vi "GPS_file_append.vi"(8 "Alt":string[](array[string]), 9 "Lng":string[](array[string]), 10 "Lat":string[](array[string]), 11 "input cluster":T1={"System"={"Active"=FALSE, "Exit"=FALSE, "Command wait"="", "Status_Time"=0, "Time_GPS"=0}, "Stepper Motor"={"Connection Reference"="", "Valid Connection"=FALSE, "Speed"=15}, "Camera Data"={"Image path"=path "", "Filenames"=[], "Filenames queue"=[]}, "Core"={"Close Panel on Exit?"=FALSE, "Current VI Reference"=refnum}} {"Stepper Motor"."Speed" scale=0.0..30.0}) -> (2 "Data":string[][](array[string]), 3 "Filenames queue":string[](array[string]))   [LabVIEW 2019]
uses:
  System Data.ctl
  Stepper Data.ctl
  Camera Data.ctl
  <vilib>/Utility/file.llb/Write Delimited Spreadsheet (string).vi
  <vilib>/Utility/file.llb/Read Delimited Spreadsheet (string).vi
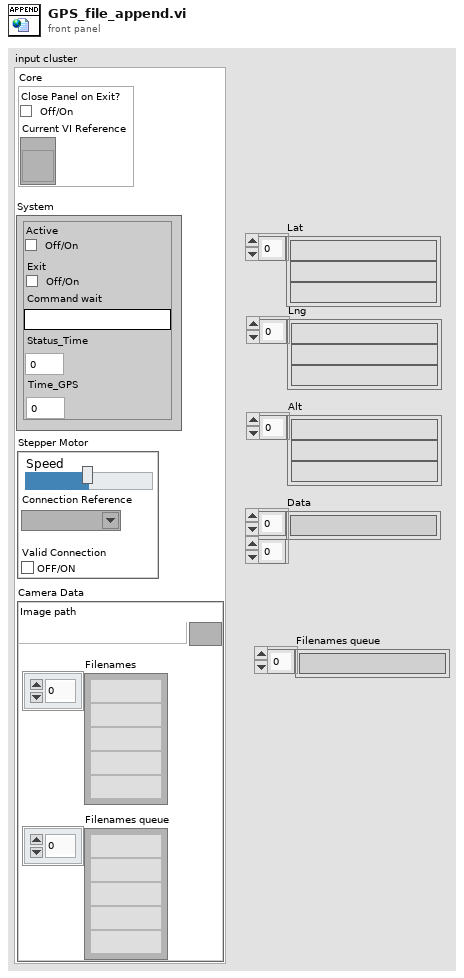
[diagram p1: front panel]
types:
  T1 = typedef "System Data.ctl" = cluster{"System":cluster{"Active":bool, "Exit":bool, "Command wait":string, "Status_Time":i32, "Time_GPS":i32}, "Stepper Motor":T2, "Camera Data":T3, "Core":cluster{"Close Panel on Exit?":bool, "Current VI Reference":refnum<vi>}}
  T2 = typedef "Stepper Data.ctl" = cluster{"Connection Reference":refnum<visa-resource-name>, "Valid Connection":bool, "Speed":i32}
  T3 = typedef "Camera Data.ctl" = cluster{"Image path":path, "Filenames":string[], "Filenames queue":string[]}
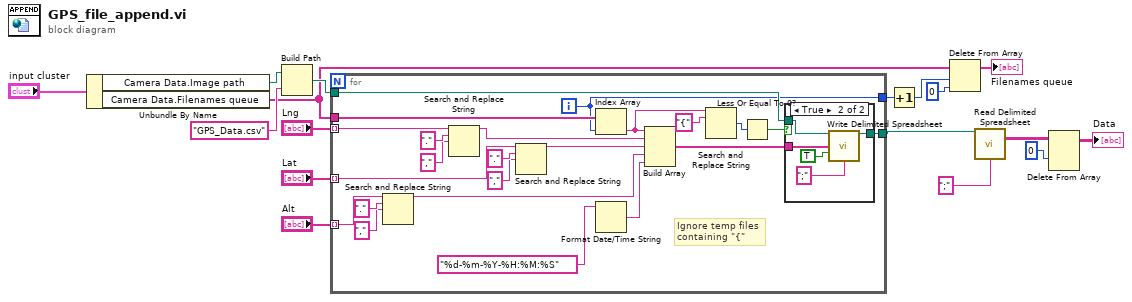
[diagram p0: block diagram]
diagram:
  n1 = Unbundle By Name("input cluster") -> ("Camera Data.Image path"=w15:path, "Camera Data.Filenames queue"=w11:string[])
  n2 = Build Path(base path=w15, name or relative path="GPS_Data.csv") -> (appended path=w16:path)
  n3 = for {
    tunnel: "Lng" -> [w33] mode=indexing
    tunnel: "Lat" -> [w28] mode=indexing
    tunnel: w16 -> [w39]
    tunnel: w11 -> [w37]
    tunnel: [w36] -> w12
    tunnel: "Alt" -> [w24] mode=indexing
    tunnel: [w18] -> w1
    i -> [w36]
    # "Ignore temp files\ncontaining \"{\""
    n4 = Search and Replace String(input string=w24, search string=".", replace string="," ("replace string (\"\")")) -> (result string=w23:string)  [unwired: 5 in, 3 out]
    n5 = Search and Replace String(input string=w33, search string=".", replace string="," ("replace string (\"\")")) -> (result string=w34:string)  [unwired: 5 in, 3 out]
    n6 = Search and Replace String(input string=w28, search string=".", replace string="," ("replace string (\"\")")) -> (result string=w27:string)  [unwired: 5 in, 3 out]
    n7 = Index Array(array=w37, index=w36) -> (element=w20:string)
    n8 = Format Date/Time String(time format string (%c)="%d-%m-%Y-%H:%M:%S") -> (date/time string=w35:string)  [unwired: 2 in]
    n9 = Build Array(w20, w34, w27, w23, w35) -> (w40:string[])
    n10 = Search and Replace String(input string=w20, search string="{") -> (number of replacements=w21:i32)  [unwired: 6 in, 3 out]
    n11 = Less Or Equal To 0?(x=w21) -> (x <= 0?=w19:bool)
    n12 = case shown="True" w19 {
      tunnel: w40 -> [_ w45]
      tunnel: w39 -> [w41 w44]
      tunnel: [w41 w42] -> w18
      frame False {
      }
      frame True {
        n13 = call-poly <vilib>:"Write Delimited Spreadsheet.vi"("file path (dialog if empty)"=w44, "1D data"=w45, "append to file? (new file:F)"=TRUE, "delimiter (\\t)"=";" ("delimiter (\\t)")) -> ("new file path (Not A Path if cancelled)"=w42:path)  [unwired: 10 in, 1 out]
      }
    }
  }
  n14 = Increment(x=w12) -> (x+1=w9:i32)
  n15 = Delete From Array(array=w11, length=w9, index=0) -> (array with subset deleted=→"Filenames queue":string[])  [unwired: 1 out]
  n16 = call-poly <vilib>:"Read Delimited Spreadsheet.vi"("file path (dialog if empty)"=w1, "delimiter (\\t)"=";" ("delimiter (\\t)")) -> ("all rows"=w4:string[][])  [unwired: 8 in, 5 out]
  n17 = Delete From Array(array=w4, index (row)=0) -> (array with subset deleted=→"Data":string[][])  [unwired: 2 in, 1 out]
